vi "SplitPlotData.vi"(11 "Value":string) -> (1 "not a number":bool, 3 "Array":dbl[](array[numeric]))   [LabVIEW 2020]
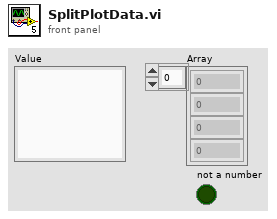
[diagram p1: front panel]
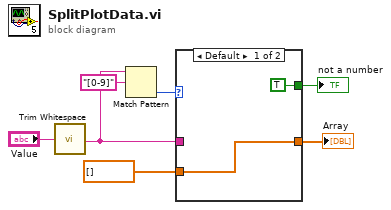
[diagram p0: block diagram]
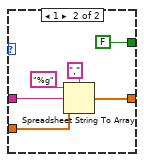
[diagram p2: hidden frame]
diagram:
  n1 = call <vilib>:"Trim Whitespace.vi"("string"="Value") -> ("trimmed string"=w4:string)  [unwired: 1 in]
  n2 = Match Pattern(string=w4, regular expression="[0-9]") -> (offset past match=w2:i32)  [unwired: 1 in, 3 out]
  n3 = case shown="Default" w2 {
    tunnel: dbl[] [] -> [w9 w14]
    tunnel: [w9 w13] -> w6
    tunnel: w4 -> [_ w11]
    tunnel: [TRUE ("not a number") FALSE ("not a number")] -> w1
    frame Default {
    }
    frame 1 {
      n4 = Spreadsheet String To Array(delimiter (Tab)=",", format string="%g", spreadsheet string=w11, array type (2D Dbl)=w14) -> (array=w13:dbl[])
    }
  }
  "Array" <- w6
  "not a number" <- w1
